vi "Create Data Message.vi"(9 "Run ID":string, 10 "Sample":T1) -> (2 "Message":string)   [LabVIEW 2024, in "Sift Client.lvlib"]
doc: "Create a serialized data message to send to Sift Proxy."
uses:
  Sift Client.lvlib
  Typedefs/Ingestion/Sample.ctl
  Typedefs/Ingestion/Timestamp.ctl
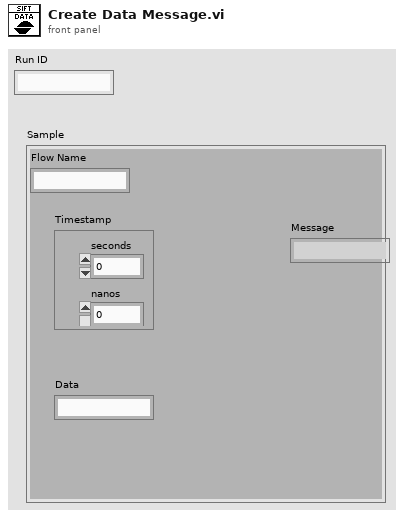
[diagram p1: front panel]
types:
  T1 = typedef "Sift Client.lvlib/Sample.ctl" = cluster{"Flow Name":string, "Timestamp":T2, "Data":string}
  T2 = typedef "Sift Client.lvlib/Timestamp.ctl" = cluster{"seconds":i64, "nanos":i32}
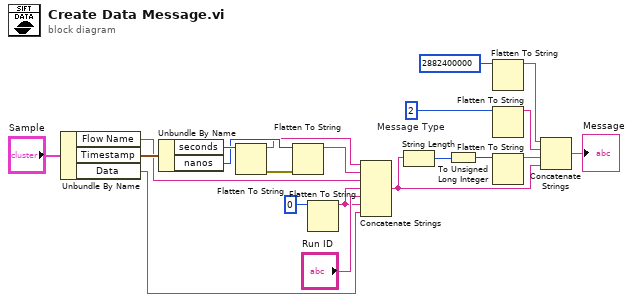
[diagram p0: block diagram]
diagram:
  w16 = u8 2  # Message Type
  n1 = Unbundle By Name("Sample") -> ("Flow Name"=w13:string, "Timestamp"=w20:T2, "Data"=w9:string)
  n2 = Unbundle By Name(w20) -> ("seconds"=w19:i64, "nanos"=w18:i32)
  n3 = Flatten To String(anything=w19) -> (data string=w15:string, error out=w17:errorcluster)  [unwired: 3 in, 1 out]
  n4 = Flatten To String(anything=w18, error in (no error)=w17) -> (data string=w14:string)  [unwired: 2 in, 2 out]
  n5 = Flatten To String(anything=u8 0) -> (data string=w10:string)  [unwired: 3 in, 2 out]
  n6 = Concatenate Strings(w15, w14, w13, w10, "Run ID", w10, w9) -> (w6:string)
  n7 = String Length(string=w6) -> (length=w2:i32)
  n8 = To Unsigned Long Integer(number=w2) -> (unsigned 32bit integer=w1:u32)
  n9 = Flatten To String(anything=u32 2882400000) -> (data string=w3:string)  [unwired: 3 in, 2 out]
  n10 = Flatten To String(anything=w16) -> (data string=w8:string)  [unwired: 3 in, 2 out]
  n11 = Flatten To String(anything=w1) -> (data string=w7:string)  [unwired: 3 in, 2 out]
  n12 = Concatenate Strings(w3, w8, w7, w6) -> (→"Message":string)
